vi "Update UI Font.vi"(8 "error in (no error)":errorcluster, 11 "dup file":path) -> (0 "error out":errorcluster, 3 "dup file (dup)":path)   [LabVIEW 2014]
uses:
  <vilib>/Utility/config.llb/Write Key (String).vi
  <vilib>/Utility/config.llb/NI_LVConfig.lvlib
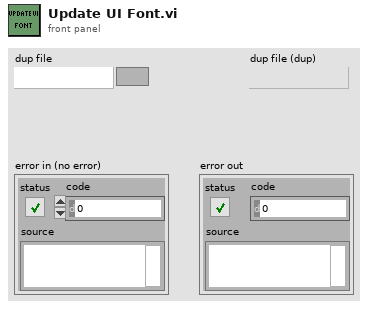
[diagram p1: front panel]
types:
  T1 = typedef "NI_LVConfig.lvlib/Config Data RefNum.ctl" = refnum<k1>
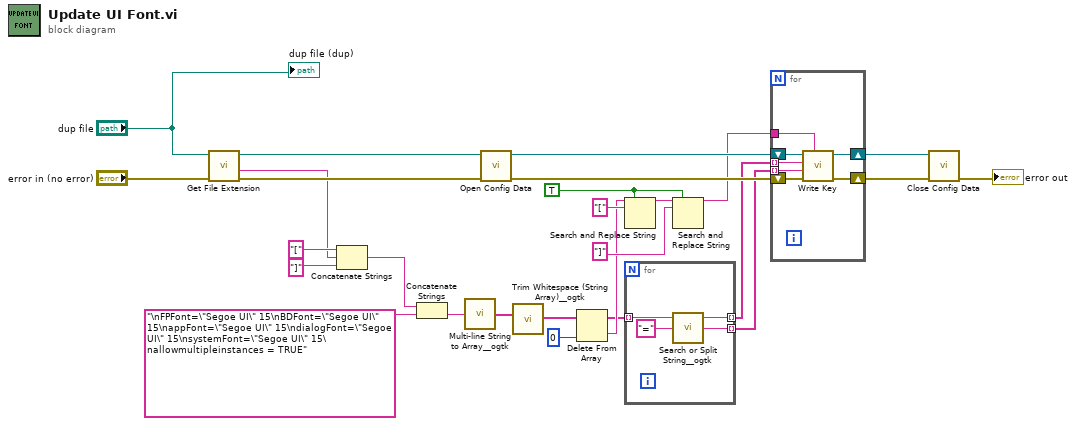
[diagram p0: block diagram]
diagram:
  w18 = TRUE ("replace all? (F)")
  n1 = call <vilib>:"Get File Extension.vi"("error in (no error)"="error in (no error)", "file"="dup file") -> ("error out"=w4:errorcluster, "filename without extension"=w3:string, "dup file"=w1:path)  [unwired: 6 in, 1 out]
  n2 = Concatenate Strings("[" ("string"), w3, "]" ("string")) -> (w27:string)
  n3 = Concatenate Strings(w27, "\nFPFont=\"Segoe UI\" 15\nBDFont=\"Segoe UI\" 15\nappFont=\"Segoe UI\" 15\ndialogFont=\"Segoe UI\" 15\nsystemFont=\"Segoe UI\" 15\nallowmultipleinstances = TRUE" ("String")) -> (w24:string)
  n4 = call <userlib>:"Multi-line String to Array__ogtk.vi"("string"=w24) -> ("lines"=w11:string[])
  n5 = call <vilib>:"Open Config Data.vi"("error in (no error)"=w4, "configuration file path"=w1) -> ("error out"=w22:errorcluster, "refnum"=w19:T1)  [unwired: 7 in, 1 out]
  n6 = call <userlib>:"Trim Whitespace (String Array)__ogtk.vi"("String in"=w11) -> ("String out"=w10:string[])  [unwired: 6 in]
  n7 = Delete From Array(array=w10, index=0) -> (deleted portion=w13:string, array with subset deleted=w8:string[])  [unwired: 1 in]
  n8 = Search and Replace String(replace all?=w18, input string=w13, search string="[") -> (result string=w15:string)  [unwired: 5 in, 3 out]
  n9 = for {
    tunnel: w8 -> [w31] mode=indexing
    tunnel: [w29] -> w7 mode=indexing
    tunnel: [w28] -> w6 mode=indexing
    n10 = call <userlib>:"Search or Split String__ogtk.vi"("search string/char (-)"="=", "string"=w31) -> ("substring after match"=w28:string, "substring before match"=w29:string)  [unwired: 1 in, 1 out]
  }
  n11 = Search and Replace String(replace all?=w18, input string=w15, search string="]") -> (result string=w14:string)  [unwired: 5 in, 3 out]
  n12 = for {
    tunnel: w14 -> [w34]
    shift-right: [w36] -> w21
    shift-left: w19 -> [w38]
    shift-right: [w35] -> w23
    shift-left: w22 -> [w37]
    tunnel: w7 -> [w33] mode=indexing
    tunnel: w6 -> [w32] mode=indexing
    n13 = call-poly <vilib>:"Write Key.vi"("section"=w34, "error in (no error)"=w37, "value"=w32, "key"=w33, "refnum"=w38) -> ("error out"=w35:errorcluster, "refnum out"=w36:T1)  [unwired: 4 in, 1 out]
  }
  n14 = call <vilib>:"Close Config Data.vi"("error in (no error)"=w23, "refnum"=w21) -> ("error out"=→"error out":errorcluster)  [unwired: 8 in, 1 out]
  "dup file (dup)" <- "dup file"
